vi "getChannel_nameXML.vi"(8 "error in (no error)":errorcluster, 11 "ScriptEvent in":refnum<class "ScriptEvent.lvclass">) -> (0 "error out":errorcluster, 2 "channel_nameXML":refnum<class "xmlNode.lvclass">, 3 "ScriptEvent out":refnum<class "ScriptEvent.lvclass">)   [LabVIEW 2009, in "Tools.lvlib" / "Scripting.lvlib" / "ScriptEvent.lvclass"]
uses:
  ScriptEvent.lvclass
  xmlNode/xmlNode.lvclass
  ScriptEvent.lvclass/ScriptEvent.ctl
  DatabaseHelpers/Database Objects/Channel/Channel.lvclass
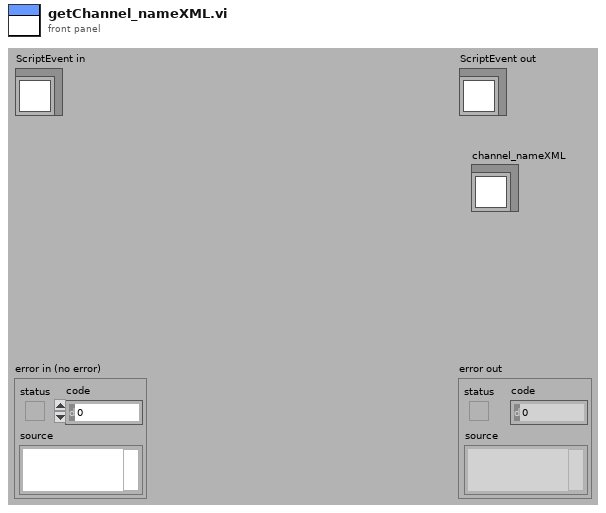
[diagram p1: front panel]
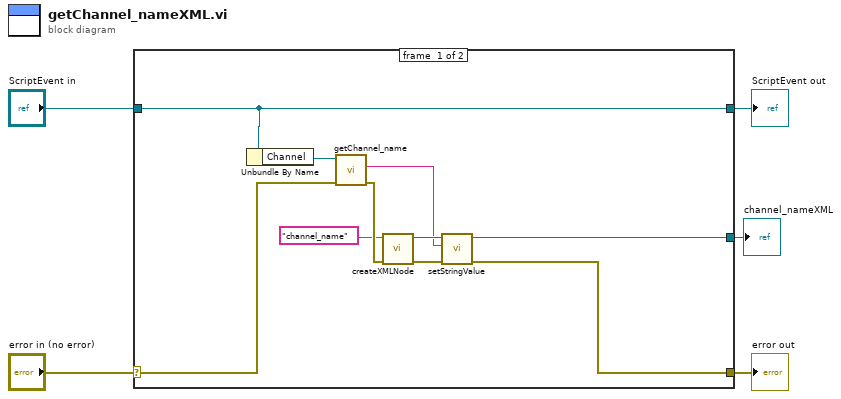
[diagram p0: block diagram]
diagram:
  n1 = case shown="No Error" "error in (no error)" {
    selector: "error in (no error)" -> [w7 w17]
    tunnel: [w6 w17] -> w4
    tunnel: [w13 w16] -> w2
    tunnel: "ScriptEvent in" -> [w13 w16]
    tunnel: [w8 _] -> w1
    frame #0 {
      n2 = Unbundle By Name(w13) -> ("Channel"=w12:refnum<class "Channel.lvclass">)
      n3 = call "getChannel_name.vi"("error in (no error)"=w7, "Channel.lvclass in"=w12) -> ("error out"=w11:errorcluster, "channel_name"=w10:string)  [unwired: 7 in, 1 out]
      n4 = call "createXMLNode.vi"("error in (no error)"=w11, "name"="channel_name") -> ("error out"=w14:errorcluster, "xmlNode out"=w15:refnum<class "xmlNode.lvclass">)  [unwired: 8 in]
      n5 = call-dynamic "setStringValue.vi"("error in (no error)"=w14, "stringValue"=w10, "xmlNode.lvclass in"=w15) -> ("error out"=w6:errorcluster, "xmlNode.lvclass out"=w8:refnum<class "xmlNode.lvclass">)  [unwired: 7 in]
    }
    frame #1 {
    }
  }
  "error out" <- w4
  "ScriptEvent out" <- w2
  "channel_nameXML" <- w1
